vi "ChannelConfigure.vi"(2 "Channel Setting 1":T1 {"Meas Range" items=["-0.1 V~+0.1 V"=0.1, "-0.2 V~0.2 V"=0.2, "-0.5 V~+0.5 V"=0.5, "-1 V~+1 V"=1.0, "-2 V~+2 V"=2.0, "-5 V~+5 V"=5.0, "-10 V~+10 V"=10.0]; "Vertical\nPosition (Div)" min=-5.0 max=5.0 step=0.01 scale=-5.0..5.0 scale format="%.2f"; "Scale\n  Volts/Div" scale=0.01..20.0}, 3 "Error In":errorcluster caption="错误输出", 4 "Channel Setting 0":T1 {"Meas Range" items=["-0.1 V~+0.1 V"=0.1, "-0.2 V~0.2 V"=0.2, "-0.5 V~+0.5 V"=0.5, "-1 V~+1 V"=1.0, "-2 V~+2 V"=2.0, "-5 V~+5 V"=5.0, "-10 V~+10 V"=10.0]; "Vertical\nPosition (Div)" min=-5.0 max=5.0 step=0.01 scale=-5.0..5.0 scale format="%.2f"; "Scale\n  Volts/Div" scale=0.01..20.0}) -> (0 "Error Out":errorcluster caption="错误输出", 1 "Task Out":refnum<k21> caption="任务输出")   [LabVIEW 2012]
uses:
  <vilib>/DAQmx/create/channels.llb/DAQmx Create Channel (AI-Voltage-Basic).vi
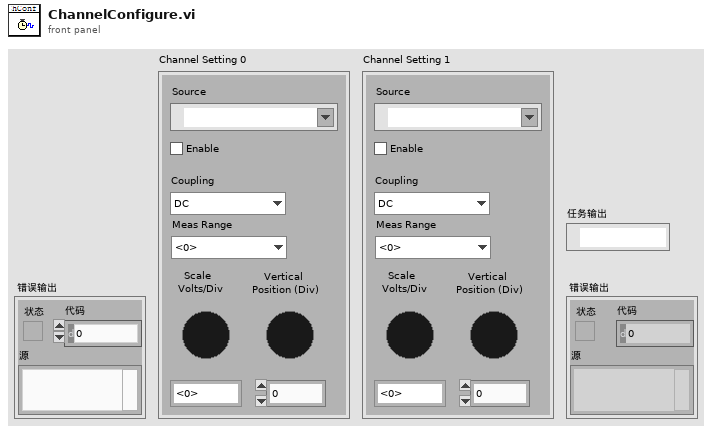
[diagram p1: front panel]
types:
  T1 = cluster{"physical channels":tag, "Enable":bool, "Coupling":enum16{"DC", "AC"}, "    Scale\n  Volts/Div  ":dbl, "    Vertical\nPosition (Div)":dbl, "Meas Range":dbl}
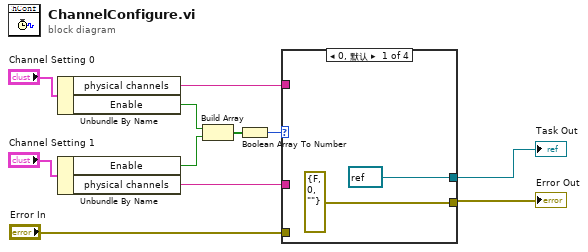
[diagram p0: block diagram]
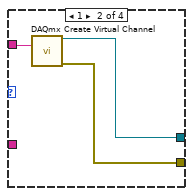
[diagram p2: hidden frame]
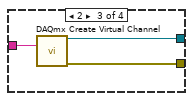
[diagram p3: hidden frame]
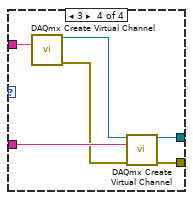
[diagram p4: hidden frame]
diagram:
  n1 = Unbundle By Name("Channel Setting 0") -> ("physical channels"=w11:tag, "Enable"=w5:bool)
  n2 = Unbundle By Name("Channel Setting 1") -> ("Enable"=w4:bool, "physical channels"=w7:tag)
  n3 = Build Array(w5, w4) -> (w3:bool[])
  n4 = Boolean Array To Number(Boolean array=w3) -> (number=w2:u32)
  n5 = case shown="0, 默认" w2 {
    tunnel: w11 -> [_ w16 _ w24]
    tunnel: w7 -> [_ _ w19 w23]
    tunnel: [refnum<k21> refnum ("task out") w15 w18 w22] -> w10
    tunnel: [errorcluster {"status"=FALSE, "code"=0, "source"=""} ("error out") w14 w17 w21] -> w6
    tunnel: "Error In" -> [_ _ _ _]
    frame 0, Default {
    }
    frame 1 {
      n6 = call-poly <vilib>:"DAQmx Create Virtual Channel.vi"("physical channels"=w16) -> ("task out"=w15:refnum<k21>, "error out"=w14:errorcluster)  [unwired: 13 in]
    }
    frame 2 {
      n7 = call-poly <vilib>:"DAQmx Create Virtual Channel.vi"("physical channels"=w19) -> ("task out"=w18:refnum<k21>, "error out"=w17:errorcluster)  [unwired: 13 in]
    }
    frame 3 {
      n8 = call-poly <vilib>:"DAQmx Create Virtual Channel.vi"("physical channels"=w24) -> ("task out"=w25:refnum<k21>, "error out"=w20:errorcluster)  [unwired: 13 in]
      n9 = call-poly <vilib>:"DAQmx Create Virtual Channel.vi"("task in"=w25, "physical channels"=w23, "error in"=w20) -> ("task out"=w22:refnum<k21>, "error out"=w21:errorcluster)  [unwired: 11 in]
    }
  }
  "Task Out" <- w10
  "Error Out" <- w6
